vi "NewAutoCorrPt.vi"(5 "Modulo":i64, 6 "Second?":bool, 7 "First?":bool, 9 "divisor":i32, 10 "AC final pts":i64, 11 "New Count":dbl) -> (1 "interation out":i64, 2 "G2 out":dbl[](array[numeric]), 3 "bin out":dbl)   [LabVIEW 2022 SP3]
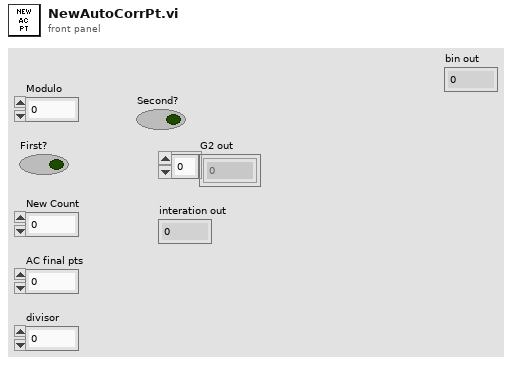
[diagram p1: front panel]
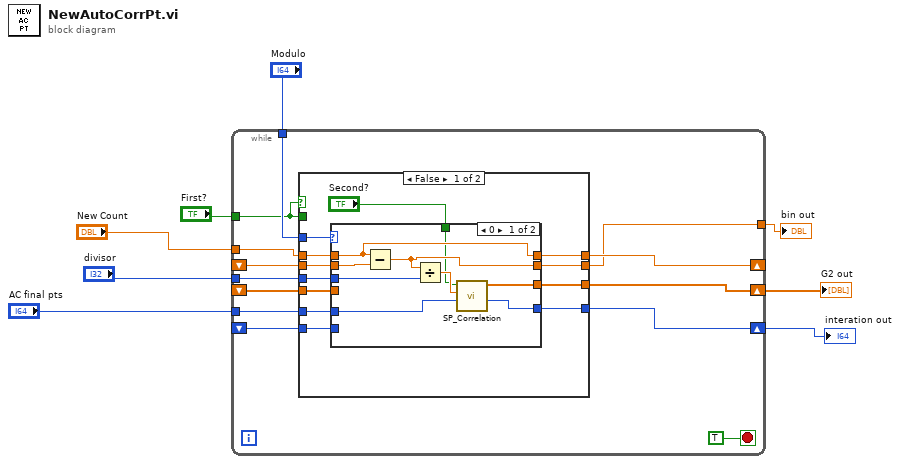
[diagram p0: block diagram]
diagram:
  n1 = while {
    tunnel: "divisor" -> [w21]
    tunnel: "First?" -> [w9]
    tunnel: "New Count" -> [w20]
    tunnel: "AC final pts" -> [w19]
    tunnel: "Modulo" -> [w13]
    shift-right: [w12] -> w2
    shift-left: _ -> [w16]
    shift-right: [w17] -> w4
    shift-left: _ -> [w18]
    shift-right: [w14] -> _
    shift-left: _ -> [w15]
    tunnel: [w10] -> w1
    stop <- TRUE stop-if-true
    n2 = case shown="False" w9 {
      tunnel: w21 -> [w33 _]
      tunnel: w20 -> [w32 w46]
      tunnel: w19 -> [w31 _]
      tunnel: w18 -> [w30 _]
      tunnel: [w29 _] -> w17
      tunnel: w16 -> [w28 _]
      tunnel: w15 -> [w27 _]
      tunnel: [w26 w46] -> w14
      tunnel: w13 -> [w25 _]
      tunnel: [w24 _] -> w12
      tunnel: [w23 _] -> w10
      tunnel: w9 -> [_ _]
      frame False {
        n3 = case shown="0" w25 {
          tunnel: w31 -> [w42 _]
          tunnel: [w41 w45] -> w24
          tunnel: w27 -> [w40 w43]
          tunnel: w32 -> [w38 _]
          tunnel: [w39 w44] -> w29
          tunnel: [w38 w43] -> w26
          tunnel: w33 -> [w37 _]
          tunnel: w28 -> [_ w45]
          tunnel: w30 -> [_ w44]
          tunnel: [w35 _] -> w23
          tunnel: "Second?" -> [w34 _]
          frame 0 {
            n4 = Subtract(x=w38, y=w40) -> (x-y=w35:dbl)
            n5 = Divide(x=w35, y=w37) -> (x/y=w36:dbl)
            n6 = call "SP_Correlation.vi"("Tau Number"=w42, "New Count"=w36, "initialize"=w34) -> ("interation"=w39:i64, "Cross Corr"=w41:dbl[])  [unwired: 7 in]
          }
          frame 1, Default {
          }
        }
      }
      frame True {
      }
    }
  }
  "interation out" <- w4
  "G2 out" <- w2
  "bin out" <- w1
